vi "Send Intake Data.vi"(10 "DVR In":refnum<data-value>) -> ()   [LabVIEW 2016]
uses:
  Intake Notifier.ctl
  Intake Control Type.ctl
  Intake Globals.vi
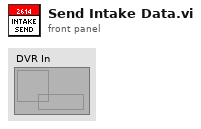
[diagram p1: front panel]
types:
  T1 = typedef "Intake Notifier.ctl" = cluster{"In":bool, "Out":bool, "Intake Control List":T2}
  T2 = typedef "Intake Control Type.ctl" = enum16{"No Op", "In", "Out"}
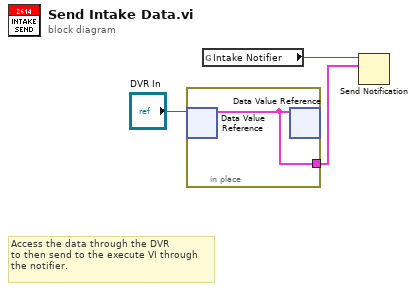
[diagram p0: block diagram]
diagram:
  # "Access the data through the DVR\nto then send to the execute VI through\nthe notifier."
  n1 = in-place {
    in-place-border: [w4] -> w2
    n2 = in-place-dvr #1("DVR In") -> (w4:T1)  [unwired: 1 out]
    n3 = in-place-dvr #1(w4) -> ()  [unwired: 2 out]
  }
  n4 = global read "Intake Globals.vi" "Intake Notifier"() -> (w1:refnum<notifier>)
  n5 = Send Notification(notification=w2, notifier=w1) -> ()  [unwired: 1 in, 2 out]
